vi "Robot Main.vi"() -> ()   [LabVIEW 2019]
uses:
  <vilib>/Rock Robotics/WPI/DriverStation/WPI_DriverStationRobotMode2.ctl
  MiscSupportPrograms/Radio_Speed_Ctrl.ctl
  ShootDualTalonSRX/Dist_Type.ctl
  ShootDualTalonSRX/Time_Units_Control.ctl
  <vilib>/Rock Robotics/WPI/Joystick/WPI_JoystickDeviceEnum.ctl
  Robot Global Data.vi
  <vilib>/Rock Robotics/WPI/Joystick/WPI_JoystickArcadeMapping.vi
  ShootDualTalonSRX/ShootDualTalonSRX_Motor_Pair.lvlib
panel:
  in  "Right Speed \nDemand\nPERCENT":T1=enum."Radio Selection 7"
  in  "Left Speed \nDemand\nPERCENT":T1=enum."Radio Selection 7"
  out "VELOCITY CTRL":bool
  in  "Tab Control":enum32{"Operation", "Left Tune", "Right Tune"}(tab)
  out "Encoder Edges Per Rev":dbl=5000.0
  in  "Encoder counts Per Rev":dbl=1024.0
  in  "Max Sped (Units)":dbl=5000.0
  out "Robot Mode":T2
  out "LeftSpeed\nTarget":dbl format="%.2f"
  out "RigthSpeed\nTarget":dbl format="%.2f"
  in  "RIght CAN":u8=14
  in  "Left CAN":u8=13
  in  "Enable \nClosed Loop":bool=TRUE
  in  "Use \nJoyStick":bool
  out "Left Speed\nRPM":dbl format="%.2f"
  out "Right Speed\nRPM":dbl format="%.2f"
  in  "Wheel Radius In":dbl=3.0 format="%.4f"
  in  "Distance Type":T3
  in  "Time":T4=enum."/ Minute"
  out "Count/Dist":dbl format="%.4f"
  out "Dist/Count":dbl format="%.4f"
  out "Units":string
  out "Count/VelUnits In 0.1 SEC":dbl format="%.4f"
  out "VelUnits/Count in 0.1":dbl format="%.4f"
  in  "update left":bool
  out "Speed Closed Loop Plots RAW L":cluster{dbl, dbl}(graph)
  out "Applied Output  L":dbl format="%.5f"
  in  "Kp L":dbl=0.01611 format="%.5f"
  in  "KI L":dbl=0.0012 format="%.5f"
  in  "Kd L":dbl=0.01 format="%.5f"
  in  "FF L":dbl=0.01611 format="%.5f"
  in  "I Zone L":dbl=600.0 format="%.5f"
  out "Encoder Velocity Units Per 100ms L":dbl format="%.5f"
  out "Target Velocity Units per 100ms L":dbl format="%.5f"
  out "Motor output Plot L":cluster{"Percent Output":dbl}(graph)
  out "Raw encoder counts  L":dbl
  out "Speed Closed Loop Plots ENG L":cluster{dbl, dbl}(graph)
  out "Speed Dmd  FT/SEC L":dbl format="%.5f"
  out "Speed  FT/SEC L":dbl format="%.5f"
  in  "F Open Loop L":dbl=0.01611 format="%.5f"
  out "Distance FT L":dbl format="%.5f"
  out "Left FF\nAdj Mult":dbl format="%.6f"
  in  "update right":bool
  out "Speed Closed Loop Plots RAW R":cluster{dbl, dbl}(graph)
  out "Applied Output R":dbl format="%.5f"
  in  "Kp R":dbl=0.01611 format="%.5f"
  in  "KI R":dbl=0.0012 format="%.5f"
  in  "Kd R":dbl=0.01 format="%.5f"
  in  "FF R":dbl=0.01611 format="%.5f"
  in  "I Zone R":dbl=600.0 format="%.5f"
  out "Encoder Velocity Units Per 100ms R":dbl format="%.5f"
  out "Target Velocity Units per 100ms R":dbl format="%.5f"
  out "Motor output Plot R":cluster{"Applied Throttle":dbl}(graph)
  out "Raw encoder counts R":dbl
  out "Speed Closed Loop Plots ENG R":cluster{dbl, dbl}(graph)
  out "Speed Dmd FT/SEC R":dbl format="%.5f"
  out "Speed FT/SEC R":dbl format="%.5f"
  in  "F Open Loop R":dbl=0.01611 format="%.5f"
  out "Distance FT R":dbl format="%.5f"
  out "Right FF\nAdj Mult":dbl format="%.6f"
  # "x"
  # "Filtered\n600 ms\naverage"
  # "Set CAN ID before\nstarting execution..."
  # "original\nf .01611\np .01611\ni .0012\nd .01"
  # "original\nf .01611\np .01611\ni .0012\nd .01"
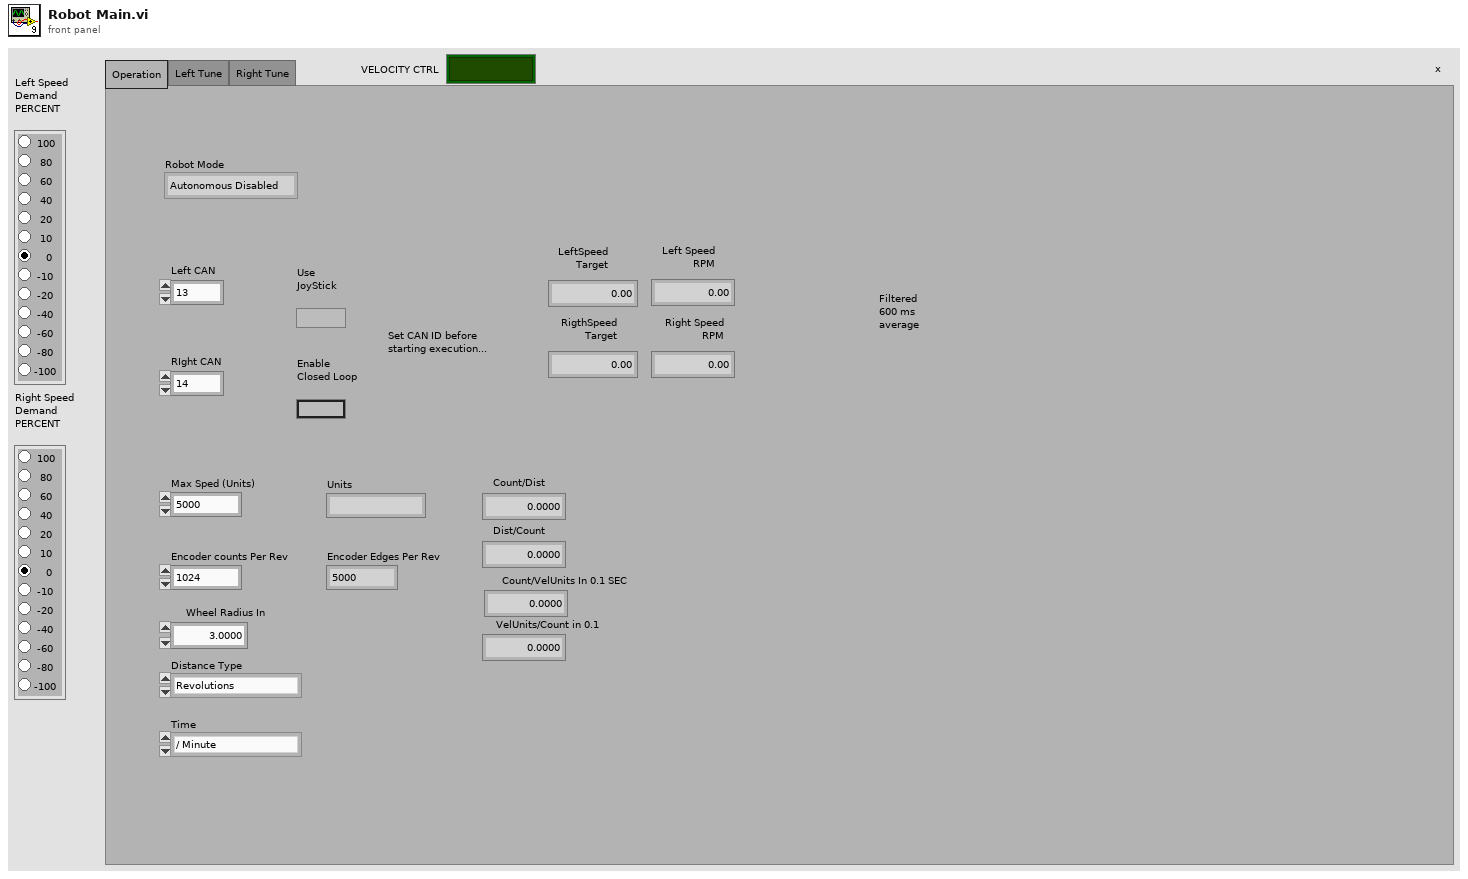
[diagram p1: front panel]
types:
  T1 = typedef "Radio_Speed_Ctrl.ctl" = enum32{"Radio Selection 1", "Radio Selection 2", "Radio Selection 3", "Radio Selection 4", "Radio Selection 5", "Radio Selection 6", "Radio Selection 7", "Radio Selection 8", "Radio Selection 9", "Radio Selection 10", "Radio Selection 11", "Radio Selection 12", "Radio Selection 13"}
  T2 = typedef "WPI_DriverStationRobotMode2.ctl" = enum16{"Autonomous Disabled", "Autonomous Enabled", "Teleop Disabled", "Teleop Enabled", "Disconnected", "Finish", "Test Disabled", "Test Enabled", "Emergency Stopped"}
  T3 = typedef "ShootDualTalonSRX_Motor_Pair.lvlib/Dist_Type.ctl" = enum16{"Revolutions", "Feet"}
  T4 = typedef "ShootDualTalonSRX_Motor_Pair.lvlib/Time_Units_Control.ctl" = enum16{"/ Second", "/ Minute"}
  T5 = typedef "WPI_JoystickDeviceEnum.ctl" = enum16{"USB 0", "USB 1", "USB 2", "USB 3", "USB 4", "USB 5"}
  T6 = typedef "WPI_JoystickDevRef.ctl" = cluster{"Device":T5}
  T7 = typedef "ShootDualTalonSRX_Motor_Pair.lvlib/ctrlRef_ShootDualTalon.ctl" = cluster{"LeftMasterDriveRef":T8, "RightMasterDriveRef":T8}
  T8 = typedef "WPI_MotorControlDeviceRef.ctl" = cluster{"DeviceStatus":errorcluster, "Type":T9, "PWM":cluster{"PWM Channel":T10, "DeadBand":T11}, "CAN":cluster{"Device Number":u8, "SetOutput VI Ref":variant, "GetOutput VI Ref":variant, "Enable VI Ref":variant, "Disable VI Ref":variant, "Data":variant}, "Invert":bool, "DIO PWM":cluster{"PWM \"Enable\" Channel":T10, "DIOChannel":T12, "PWM Rate":dbl}}
  T9 = typedef "WPI_MotorControlType.ctl" = enum16{"PWM", "CAN", "DIO PWM"}
  T10 = typedef "FPGA_DIOPWMChannel.ctl" = enum8{"PWM 0", "PWM 1", "PWM 2", "PWM 3", "PWM 4", "PWM 5", "PWM 6", "PWM 7", "PWM 8", "PWM 9", "PWM MXP 0", "PWM MXP 1", "PWM MXP 2", "PWM MXP 3", "PWM MXP 4", "PWM MXP 5", "PWM MXP 6", "PWM MXP 7", "PWM MXP 8", "PWM MXP 9", "Invalid"}
  T11 = typedef "WPI_PWMDeadband.ctl" = cluster{"Name":string, "maxPositivePwm":i32, "minPositivePwm":i32, "centerPwm":i32, "maxNegativePwm":i32, "minNegativePwm":i32, "angularRange":u16}
  T12 = typedef "FPGA_DIOChannel.ctl" = enum8{"DIO 0", "DIO 1", "DIO 2", "DIO 3", "DIO 4", "DIO 5", "DIO 6", "DIO 7", "DIO 8", "DIO 9", "DIO MXP 0", "DIO MXP 1", "DIO MXP 2", "DIO MXP 3", "DIO MXP 4", "DIO MXP 5", "DIO MXP 6", "DIO MXP 7", "DIO MXP 8", "DIO MXP 9", "DIO MXP 10", "DIO MXP 11", "DIO MXP 12", "DIO MXP 13", "DIO MXP 14", "DIO MXP 15", "SPI Port CS1", "SPI Port CS2", "SPI Port CS3", "SPI Port MISO", "SPI Port MOSI", "Invalid"}
  T13 = cluster{"Speed Dmd  FT/SEC L":dbl, "Speed  FT/SEC L":dbl}
  T14 = cluster{"Target Velocity Units per 100ms L":dbl, "Encoder Velocity Units Per 100ms L":dbl}
  T15 = cluster{"Target Velocity Units in 100ms R":dbl, "Encoder Velocity Units in 100ms R":dbl}
  T16 = cluster{"Speed Dmd FT/SEC R":dbl, "Speed FT/SEC R":dbl}
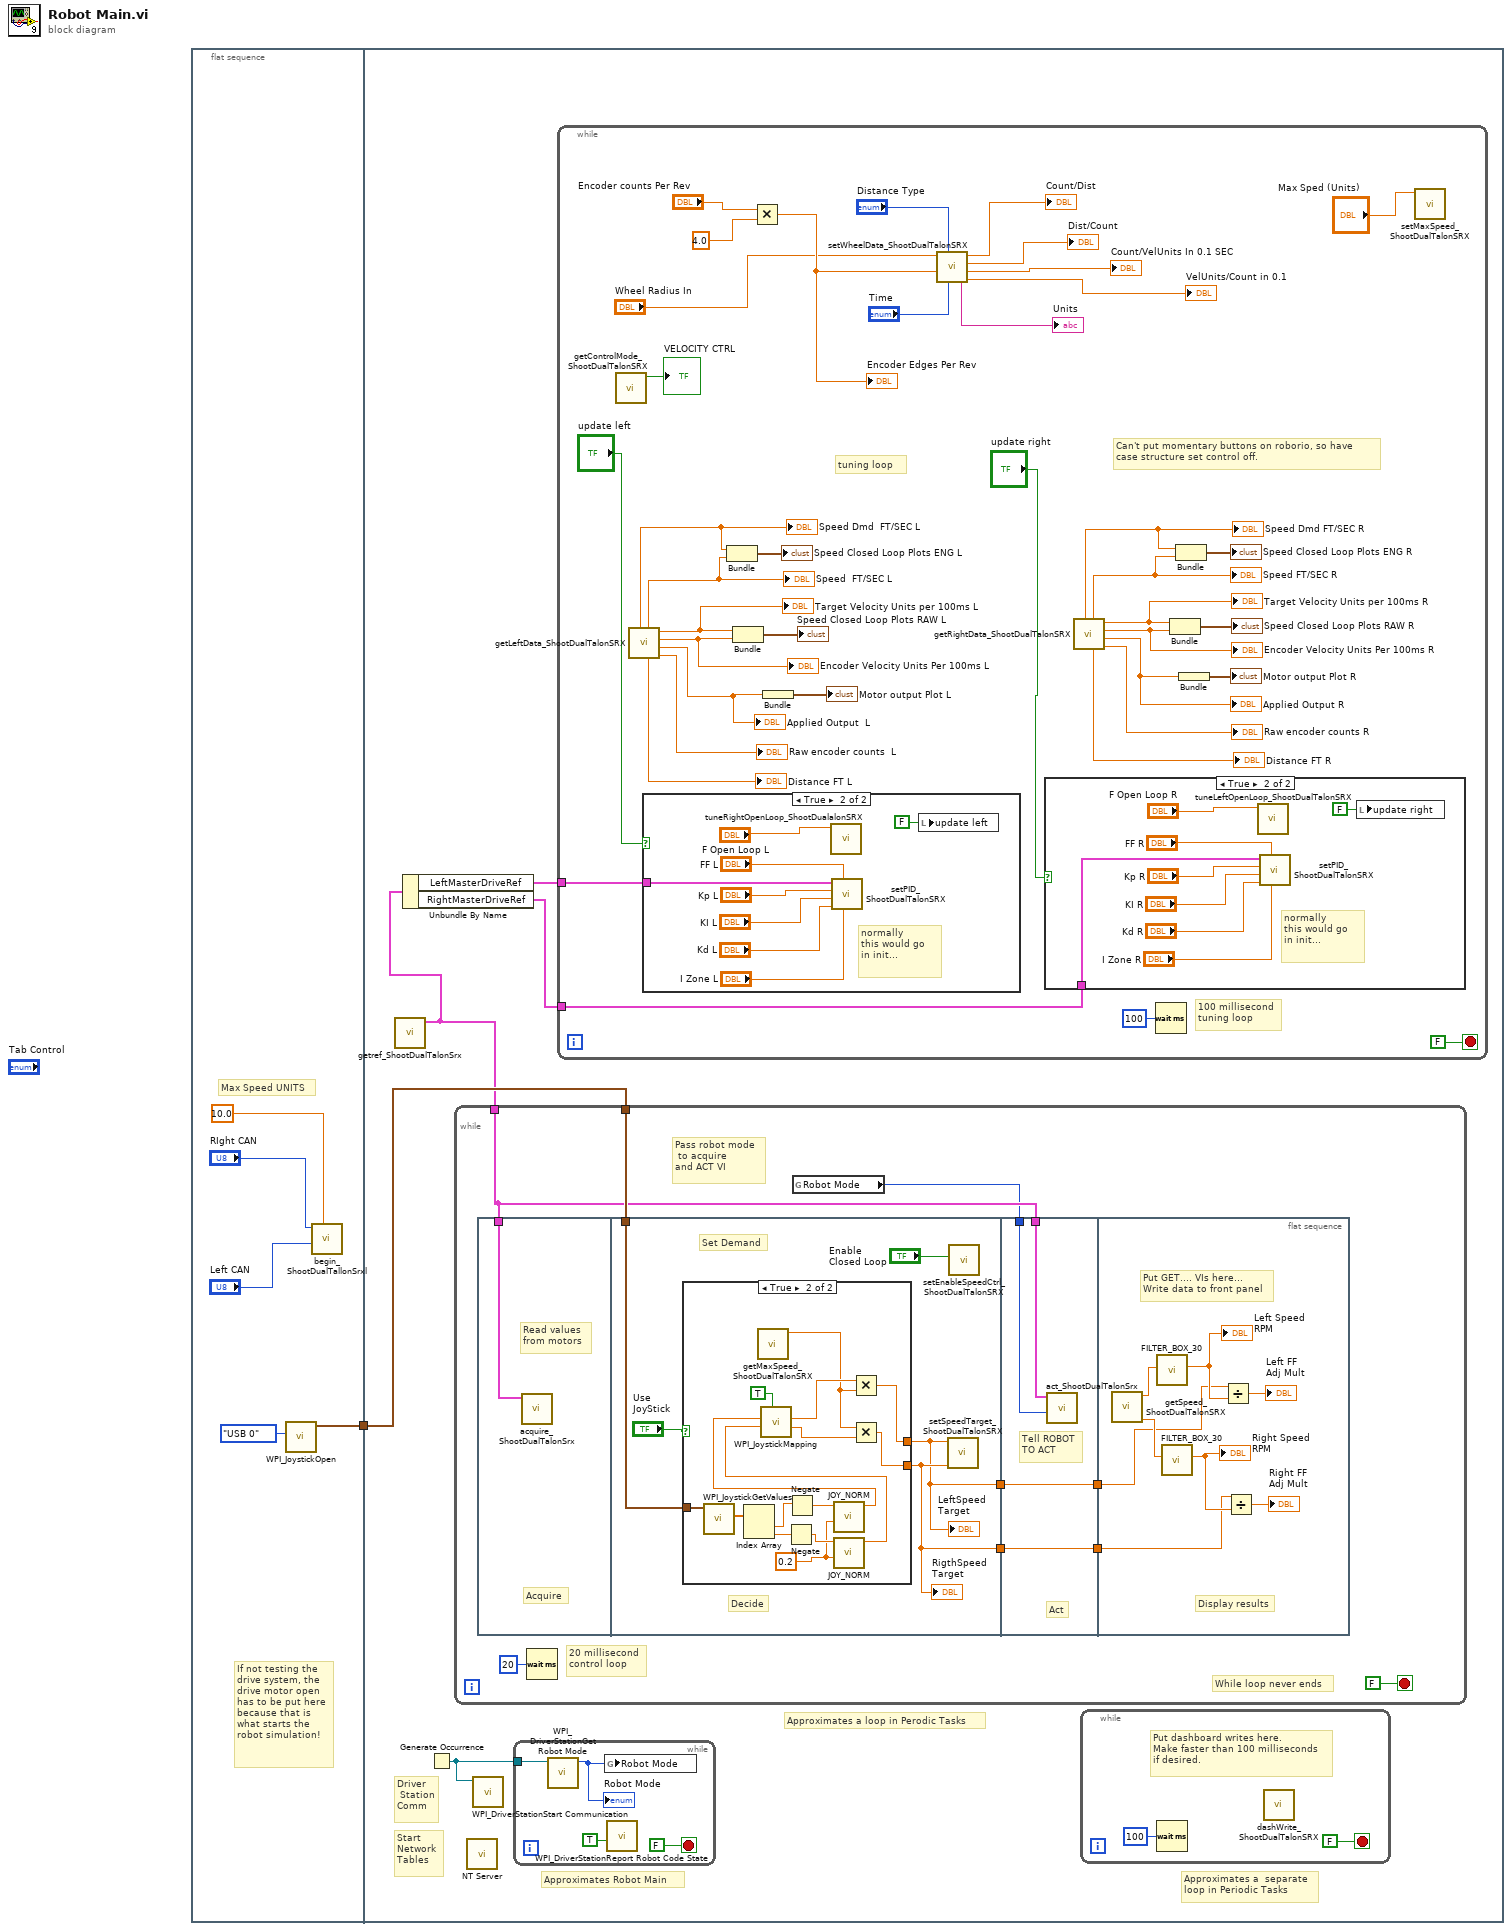
[diagram p0: block diagram]
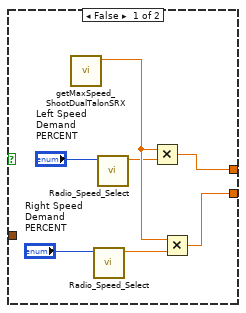
[diagram p4: hidden frame]
diagram:
  n1 = flat-sequence {
    tunnel: [w5] -> w1
    tunnel: w1 -> [w10]
    frame #0 {
      # "Max Speed UNITS"
      # "If not testing the\ndrive system, the\ndrive motor open\nhas to be put here\nbecause that is \nwhat starts the\nrobot simulation!"
      n2 = call <vilib>:"WPI_JoystickOpen.vi"("JoystickDevice"=WPI_JoystickDeviceEnum."USB 0") -> ("JoystickDevRef"=w5:T6)  [unwired: 10 in]
      n3 = call "begin_ShootDualTallonSrxl.vi"("MAX DESIRED\nVELOCITY\n(UNITS)"=10.0 ("MAX DESIRED\nVELOCITY\n(UNITS)"), "Left Master CAN"="Left CAN", "RIght Master CAN"="RIght CAN") -> ()  [unwired: 9 in]
    }
    frame #1 {
      # "Approximates a  separate\nloop in Periodic Tasks"
      # "Approximates a loop in Perodic Tasks"
      # "Approximates Robot Main"
      # "Start\nNetwork\nTables"
      # "Driver\n Station\nComm"
      n4 = call "getref_ShootDualTalonSrx.vi"() -> ("DriveRef"=w9:T7)  [unwired: 11 in]
      n5 = Unbundle By Name(w9) -> ("LeftMasterDriveRef"=w8:T8, "RightMasterDriveRef"=w7:T8)
      n6 = Generate Occurrence() -> (w11:refnum<k4>)
      n7 = while {
        tunnel: w10 -> [w79]
        tunnel: w9 -> [w78]
        stop <- FALSE stop-if-true
        # "While loop never ends"
        # "Pass robot mode\n to acquire\nand ACT VI"
        # "20 millisecond\ncontrol loop"
        n8 = flat-sequence {
          tunnel: w78 -> [w82]
          tunnel: w79 -> [w87]
          tunnel: [w84] -> w75
          tunnel: [w83] -> w73
          tunnel: w78 -> [w113]
          tunnel: w77 -> [w112]
          tunnel: [w111] -> w76
          tunnel: w75 -> [w111]
          tunnel: [w110] -> w74
          tunnel: w73 -> [w110]
          tunnel: w76 -> [w117]
          tunnel: w74 -> [w116]
          frame #0 {
            # "Read values\nfrom motors"
            # "Acquire"
            n9 = call "acquire_ShootDualTalonSrx.vi"("QuadTalonSRXDriveRef"=w82) -> ()  [unwired: 10 in, 1 out]
          }
          frame #1 {
            # "Set Demand"
            # "Decide"
            n10 = case shown="True" "Use \nJoyStick" {
              tunnel: w87 -> [_ w104]
              tunnel: [w89 w101] -> w83
              tunnel: [w88 w103] -> w84
              frame False {
                n11 = call "getMaxSpeed_ShootDualTalonSRX.vi"() -> ("Max Speed"=w92:dbl)  [unwired: 9 in, 1 out]
                n12 = call "Radio_Speed_Select.vi"("Left Speed \nDemand\nPERCENT"="Right Speed \nDemand\nPERCENT") -> ("PERCENT"=w90:dbl)  [unwired: 10 in]
                n13 = call "Radio_Speed_Select.vi"("Left Speed \nDemand\nPERCENT"="Left Speed \nDemand\nPERCENT") -> ("PERCENT"=w91:dbl)  [unwired: 10 in]
                n14 = Multiply(x=w92, y=w91) -> (x*y=w89:dbl)
                n15 = Multiply(x=w92, y=w90) -> (x*y=w88:dbl)
              }
              frame True {
                w98 = 0.2 ("Deadband")
                n16 = call <vilib>:"WPI_JoystickGetValues.vi"("JoystickDevRef"=w104) -> ("Axes"=w109:dbl[])  [unwired: 6 in, 4 out]
                n17 = Index Array(array=w109) -> (element #1=w107:dbl, element #2=w108:dbl)  [unwired: 2 in]
                n18 = call "getMaxSpeed_ShootDualTalonSRX.vi"() -> ("Max Speed"=w95:dbl)  [unwired: 9 in, 1 out]
                n19 = Negate(x=w108) -> (-x=w99:dbl)
                n20 = Negate(x=w107) -> (-x=w100:dbl)
                n21 = call "JOY_NORM.vi"("Deadband"=w98, "Joy Input"=w100) -> ("Joy Output"=w97:dbl)  [unwired: 9 in]
                n22 = call "JOY_NORM.vi"("Deadband"=w98, "Joy Input"=w99) -> ("Joy Output"=w96:dbl)  [unwired: 9 in]
                n23 = call-poly <vilib>:"WPI_JoystickMapping.vi"("Square Inputs"=TRUE, "Y axis value"=w96, "X axis value"=w97) -> ("Right Motor Value"=w102:dbl, "Left Motor Value"=w105:dbl)  [unwired: 7 in]
                n24 = Multiply(x=w105, y=w95) -> (x*y=w101:dbl)
                n25 = Multiply(x=w95, y=w102) -> (x*y=w103:dbl)
              }
            }
            "RigthSpeed\nTarget" <- w84
            "LeftSpeed\nTarget" <- w83
            n26 = call "setSpeedTarget_ShootDualTalonSRX.vi"("Right Speed Target\nFt/SEC"=w84, "Left Speed Target\nFT/SEC"=w83) -> ()  [unwired: 9 in]
            n27 = call "setEnableSpeedCtrl_ShootDualTalonSRX.vi"("Enable Speed Control"="Enable \nClosed Loop") -> ()  [unwired: 10 in]
          }
          frame #2 {
            # "Tell ROBOT\nTO ACT"
            # "Act"
            n28 = call "act_ShootDualTalonSrx.vi"("Robot Mode"=w112, "QuadTalonSRXDriveRef"=w113) -> ()  [unwired: 9 in, 1 out]
          }
          frame #3 {
            # "Put GET.... VIs here...  \nWrite data to front panel"
            # "Display results"
            n29 = call "getSpeed_ShootDualTalonSRX.vi"() -> ("Right Speed Ft/SEC"=w120:dbl, "Left Speed FT/SEC"=w121:dbl)  [unwired: 9 in]
            n30 = call "FILTER_BOX_30.vi"("Input"=w121) -> ("Filtered_Value"=w119:dbl)  [unwired: 10 in]
            "Left Speed\nRPM" <- w119
            n31 = call "FILTER_BOX_30.vi"("Input"=w120) -> ("Filtered_Value"=w118:dbl)  [unwired: 10 in]
            "Right Speed\nRPM" <- w118
            n32 = Divide(x=w116, y=w119) -> (x/y=→"Left FF\nAdj Mult":dbl)
            n33 = Divide(x=w117, y=w118) -> (x/y=→"Right FF\nAdj Mult":dbl)
          }
        }
        n34 = Wait (ms)(milliseconds to wait=u32 20) -> ()  [unwired: 1 out]
        n35 = global read "Robot Global Data.vi" "Robot Mode"() -> (w77:T2)
      }
      n36 = call <vilib>:"NT Server.vi"() -> ()  [unwired: 12 in]
      n37 = call <vilib>:"WPI_DriverStationStart Communication.vi"("occurrence"=w11) -> ()  [unwired: 11 in]
      n38 = while {
        tunnel: w11 -> [w72]
        stop <- FALSE stop-if-true
        n39 = call <vilib>:"WPI_DriverStationGet Robot Mode.vi"("DS Occurrence"=w72) -> ("Robot Mode"=w69:T2)  [unwired: 1 in, 9 out]
        "Robot Mode" <- w69
        n40 = global write "Robot Global Data.vi" "Robot Mode"(w69) -> ()
        n41 = call <vilib>:"WPI_DriverStationReport Robot Code State.vi"("TeleOp"=TRUE ("Autonomous")) -> ()  [unwired: 10 in, 1 out]
      }
      n42 = while {
        tunnel: w8 -> [w48]
        tunnel: w7 -> [w47]
        stop <- FALSE stop-if-true
        # "Can't put momentary buttons on roborio, so have\ncase structure set control off."
        # "tuning loop"
        # "100 millisecond\ntuning loop"
        n43 = call "getControlMode_ShootDualTalonSRX.vi"() -> ("VELOCITY CTRL"=→"VELOCITY CTRL":bool)  [unwired: 11 in]
        n44 = call "getLeftData_ShootDualTalonSRX.vi"() -> ("Raw encoder counts  L"=→"Raw encoder counts  L":dbl, "Applied Output  L"=w39:dbl, "Encoder Velocity Units Per 100ms L"=w40:dbl, "Target Velocity Units per 100ms L"=w41:dbl, "Distance FT L"=→"Distance FT L":dbl, "Speed  FT/SEC L"=w42:dbl, "Speed Dmd  FT/SEC L"=w36:dbl)  [unwired: 5 in]
        "Applied Output  L" <- w39
        "Encoder Velocity Units Per 100ms L" <- w40
        "Target Velocity Units per 100ms L" <- w41
        "Speed Dmd  FT/SEC L" <- w36
        "Speed  FT/SEC L" <- w42
        n45 = case shown="True" "update left" {
          tunnel: w48 -> [_ w66]
          frame False {
          }
          frame True {
            # "normally\nthis would go\nin init..."
            n46 = call "tuneRightOpenLoop_ShootDualalonSRX.vi"("F Open Loop L"="F Open Loop L") -> ()  [unwired: 11 in]
            n47 = call "setPID_ShootDualTalonSRX.vi"("I ZONE"="I Zone L", "FF"="FF L", "KD"="Kd L", "KI"="KI L", "KP"="Kp L", "MasterDriveRef"=w66) -> ()  [unwired: 6 in]
            n48 = local write "update left"(FALSE ("update left")) -> ()
          }
        }
        n49 = Bundle("Speed Dmd  FT/SEC L"=w36, "Speed  FT/SEC L"=w42) -> (→"Speed Closed Loop Plots ENG L":T13)  [unwired: 1 in]
        n50 = Bundle("Target Velocity Units per 100ms L"=w41, "Encoder Velocity Units Per 100ms L"=w40) -> (→"Speed Closed Loop Plots RAW L":T14)  [unwired: 1 in]
        n51 = Multiply(x="Encoder counts Per Rev", y=4.0) -> (x*y=w20:dbl)
        "Encoder Edges Per Rev" <- w20
        n52 = Bundle("Applied Output  L"=w39) -> (→"Motor output Plot L":cluster{"Applied Output  L":dbl})  [unwired: 1 in]
        n53 = call "setWheelData_ShootDualTalonSRX.vi"("Time"="Time", "Distance Type"="Distance Type", "Enc Edges / Rev"=w20, "Wheel Radius In"="Wheel Radius In") -> ("VelUnits/Count in 0.1"=→"VelUnits/Count in 0.1":dbl, "Count/VelUnits In 0.1 SEC"=→"Count/VelUnits In 0.1 SEC":dbl, "Dist/Count"=→"Dist/Count":dbl, "Count/Dist"=→"Count/Dist":dbl, "Units"=→"Units":string)  [unwired: 3 in]
        n54 = case shown="True" "update right" {
          tunnel: w47 -> [_ w58]
          frame False {
          }
          frame True {
            # "normally\nthis would go\nin init..."
            n55 = call "tuneLeftOpenLoop_ShootDualTalonSRX.vi"("F Open Loop R"="F Open Loop R") -> ()  [unwired: 11 in]
            n56 = call "setPID_ShootDualTalonSRX.vi"("I ZONE"="I Zone R", "FF"="FF R", "KD"="Kd R", "KI"="KI R", "KP"="Kp R", "MasterDriveRef"=w58) -> ()  [unwired: 6 in]
            n57 = local write "update right"(FALSE ("update right")) -> ()
          }
        }
        n58 = call "getRightData_ShootDualTalonSRX.vi"() -> ("Raw encoder counts R"=→"Raw encoder counts R":dbl, "Applied Output R"=w28:dbl, "Encoder Velocity Units in 100ms R"=w30:dbl, "Target Velocity Units in 100ms R"=w31:dbl, "Distance FT R"=→"Distance FT R":dbl, "Speed FT/SEC R"=w26:dbl, "Speed Dmd FT/SEC R"=w25:dbl)  [unwired: 5 in]
        "Applied Output R" <- w28
        "Encoder Velocity Units Per 100ms R" <- w30
        "Target Velocity Units per 100ms R" <- w31
        "Speed Dmd FT/SEC R" <- w25
        "Speed FT/SEC R" <- w26
        n59 = Wait (ms)(milliseconds to wait=u32 100) -> ()  [unwired: 1 out]
        n60 = Bundle("Target Velocity Units in 100ms R"=w31, "Encoder Velocity Units in 100ms R"=w30) -> (→"Speed Closed Loop Plots RAW R":T15)  [unwired: 1 in]
        n61 = Bundle("Speed Dmd FT/SEC R"=w25, "Speed FT/SEC R"=w26) -> (→"Speed Closed Loop Plots ENG R":T16)  [unwired: 1 in]
        n62 = Bundle("Applied Output R"=w28) -> (→"Motor output Plot R":cluster{"Applied Output R":dbl})  [unwired: 1 in]
        n63 = call "setMaxSpeed_ShootDualTalonSRX.vi"("MAX DESIRED\nVELOCITY (UNITS)"="Max Sped (Units)") -> ()  [unwired: 8 in, 2 out]
      }
      n64 = while {
        stop <- FALSE stop-if-true
        # "Put dashboard writes here.\nMake faster than 100 milliseconds\nif desired."
        n65 = Wait (ms)(milliseconds to wait=u32 100) -> ()  [unwired: 1 out]
        n66 = call "dashWrite_ShootDualTalonSRX.vi"() -> ()  [unwired: 12 in]
      }
    }
  }
